vi "BM_electrochem_cell_rinse_cycle_subVI_v2.vi"(0 "Sample Volume":dbl=10.0, 1 "Pump Parameters":T1={"Speed 1"="150", "Speed 2"="250", "Speed 3"="450", "Speed 4"="250", "UW/Sample"="5", "Sparge"="2", "Std"="4", "Waste"="15", "Air"="14", "Milli-Q"="1", "H2SO4"="6", "NaOH"="3", "Catalyst"="7", "Cell (H+ side)"="8", "Cell (sample side)"="9", "NaCl"="11"}, 5 "N cell rinses":i32=3, 7 "N syringe rinses":i32=3, 9 "Extra Milli-Q (ml)":dbl=2.0, 11 "step to ml":dbl=1920.0, 12 "COM Port":refnum<visa-resource-name>="COM12", 14 "Total Vol. (mL)":dbl=12.0) -> ()   [LabVIEW 2021]
panel:
  out "Full Command":string="V450O1P38400O15D38400"
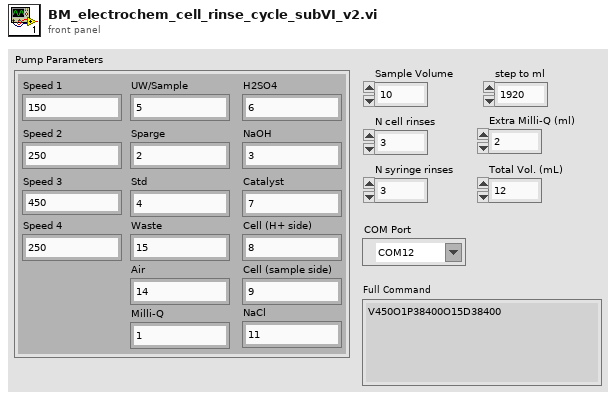
[diagram p1: front panel]
types:
  T1 = cluster{"Speed 1":string, "Speed 2":string, "Speed 3":string, "Speed 4":string, "UW/Sample":string, "Sparge":string, "Std":string, "Waste":string, "Air":string, "Milli-Q":string, "H2SO4":string, "NaOH":string, "Catalyst":string, "Cell (H+ side)":string, "Cell (sample side)":string, "NaCl":string}
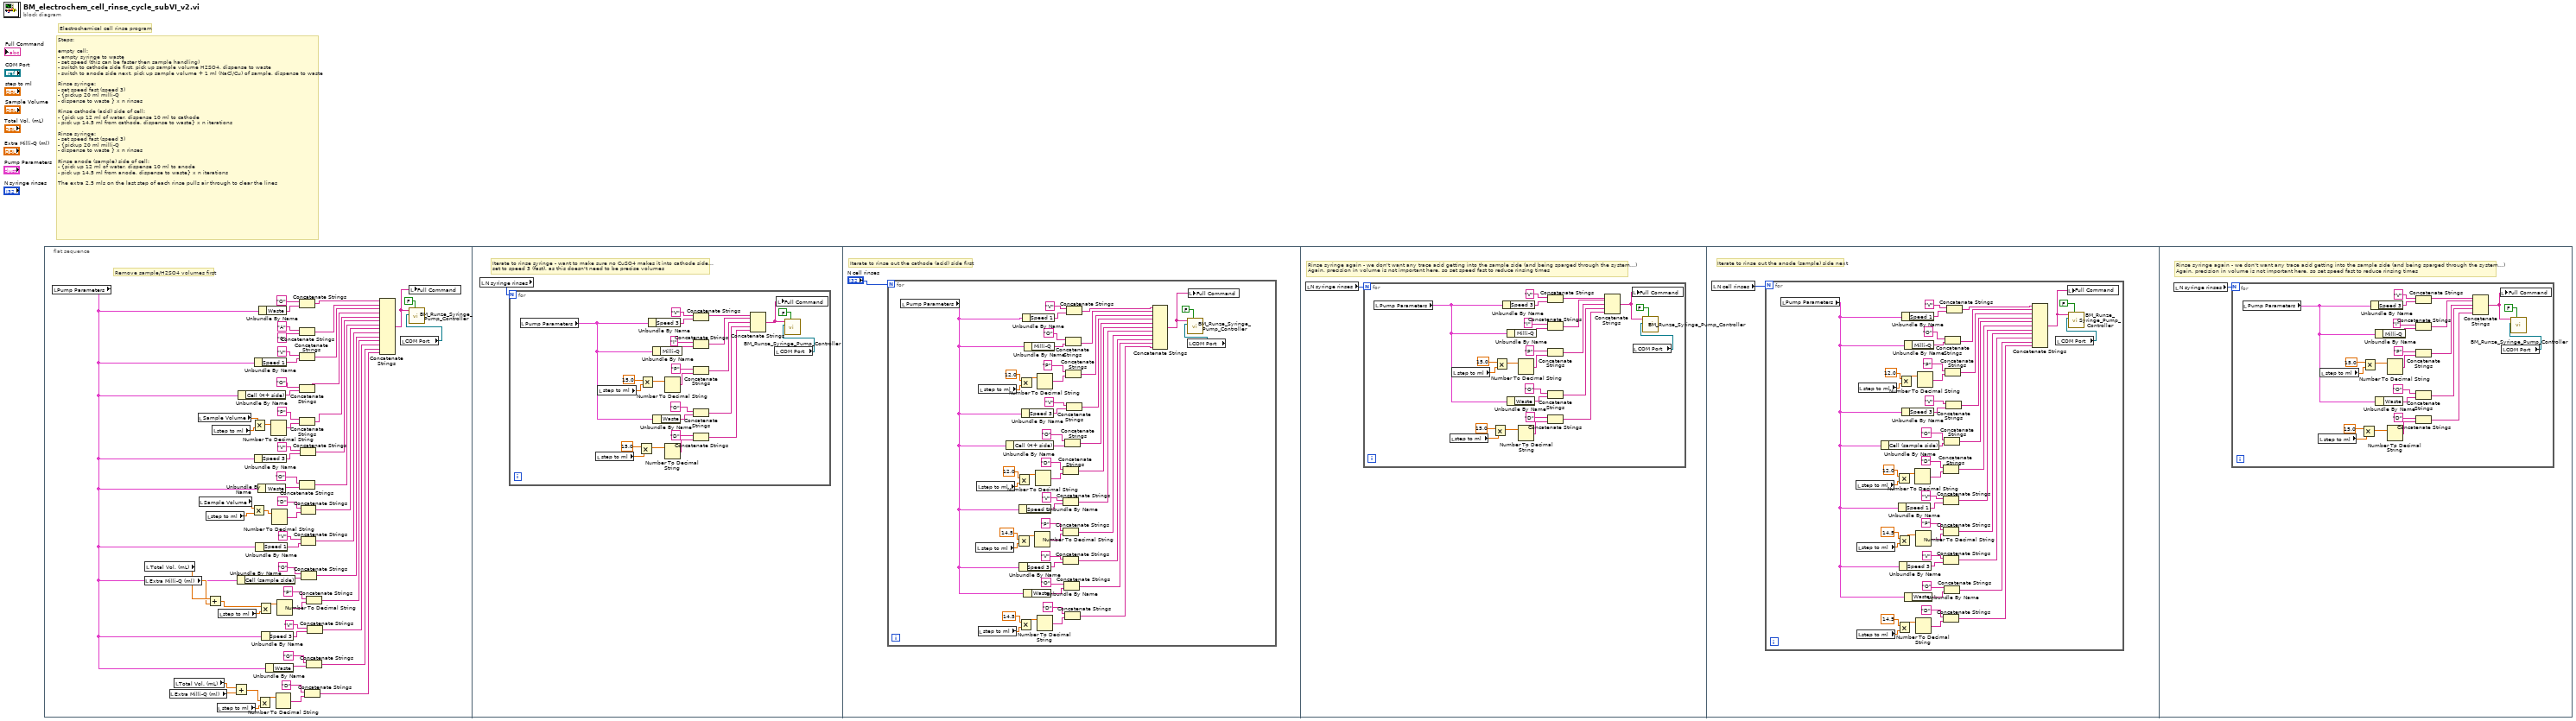
[diagram p0: block diagram]
diagram:
  # "Steps:\n\nempty cell:\n- empty syringe to waste\n- set speed (this can be faster then sample handling)\n- switch to cathode side first, pick up sample volume H2SO4, dispense to waste\n- switch to anode side next, pick up sample volume + 1 ml (NaCl/Cu) of sample, dispense to waste\n\nRinse syringe:\n- set speed fast (speed 3)\n- {pickup 20 ml milli-Q\n- dispense to waste } x n rinses\n\nRinse cathode (acid) side of cell:\n- {pick up 12 ml of water, dispense 10 ml to cathode\n- pick up 14.5 ml from cathode, dispense to waste} x n iterations\n\nRinse syringe:\n- set speed fast (speed 3)\n- {pickup 20 ml milli-Q\n- dispense to waste } x n rinses\n\nRinse anode (sample) side of cell:\n- {pick up 12 ml of water, dispense 10 ml to anode\n- pick up 14.5 ml from anode, dispense to waste} x n iterations\n\nThe extra 2.5 mls on the last step of each rinse pulls air through to clear the lines"
  # "Electrochemical cell rinse program"
  n1 = flat-sequence {
    frame #0 {
      # "Remove sample/H2SO4 volumes first"
      n2 = local read "Pump Parameters"() -> (w1:T1)
      n3 = local read "Extra Milli-Q (ml)"() -> (w30:dbl)
      n4 = local read "Total Vol. (mL)"() -> (w31:dbl)
      n5 = local read "Extra Milli-Q (ml)"() -> (w29:dbl)
      n6 = local read "Total Vol. (mL)"() -> (w19:dbl)
      n7 = local read "Sample Volume"() -> (w56:dbl)
      n8 = local read "Sample Volume"() -> (w21:dbl)
      n9 = local read "step to ml"() -> (w22:dbl)
      n10 = Add(x=w31, y=w30) -> (x+y=w27:dbl)
      n11 = local read "step to ml"() -> (w57:dbl)
      n12 = local read "step to ml"() -> (w52:dbl)
      n13 = local read "step to ml"() -> (w54:dbl)
      n14 = Add(x=w19, y=w29) -> (x+y=w18:dbl)
      n15 = Unbundle By Name(w1) -> ("Cell (sample side)"=w45:string)
      n16 = Unbundle By Name(w1) -> ("Cell (H+ side)"=w49:string)
      n17 = Multiply(x=w21, y=w22) -> (x*y=w20:dbl)
      n18 = Multiply(x=w56, y=w57) -> (x*y=w58:dbl)
      n19 = Unbundle By Name(w1) -> ("Speed 1"=w17:string)
      n20 = Unbundle By Name(w1) -> ("Speed 3"=w15:string)
      n21 = Unbundle By Name(w1) -> ("Speed 1"=w13:string)
      n22 = Multiply(x=w18, y=w52) -> (x*y=w53:dbl)
      n23 = Unbundle By Name(w1) -> ("Waste"=w25:string)
      n24 = Multiply(x=w27, y=w54) -> (x*y=w55:dbl)
      n25 = Unbundle By Name(w1) -> ("Waste"=w61:string)
      n26 = Unbundle By Name(w1) -> ("Speed 3"=w11:string)
      n27 = Unbundle By Name(w1) -> ("Waste"=w41:string)
      n28 = Number To Decimal String(number=w58) -> (decimal integer string=w47:string)  [unwired: 1 out]
      n29 = Number To Decimal String(number=w20) -> (decimal integer string=w23:string)  [unwired: 1 out]
      n30 = Number To Decimal String(number=w53) -> (decimal integer string=w39:string)  [unwired: 1 out]
      n31 = Number To Decimal String(number=w55) -> (decimal integer string=w43:string)  [unwired: 1 out]
      n32 = Concatenate Strings("O", w25) -> (w9:string)
      n33 = Concatenate Strings("O", w61) -> (w38:string)
      n34 = Concatenate Strings("A", "0") -> (w37:string)
      n35 = Concatenate Strings("V", w17) -> (w36:string)
      n36 = Concatenate Strings("O", w49) -> (w35:string)
      n37 = Concatenate Strings("P", w47) -> (w34:string)
      n38 = Concatenate Strings("V", w15) -> (w10:string)
      n39 = Concatenate Strings("D", w23) -> (w8:string)
      n40 = Concatenate Strings("V", w13) -> (w7:string)
      n41 = Concatenate Strings("O", w45) -> (w6:string)
      n42 = Concatenate Strings("D", w39) -> (w2:string)
      n43 = Concatenate Strings("P", w43) -> (w5:string)
      n44 = Concatenate Strings("O", w41) -> (w3:string)
      n45 = Concatenate Strings("V", w11) -> (w4:string)
      n46 = Concatenate Strings(w38, w37, w36, w35, w34, w10, w9, w8, w7, w6, w5, w4, w3, w2) -> (w33:string)
      n47 = local read "COM Port"() -> (w32:refnum<visa-resource-name>)
      n48 = call "BM_Runze_Syringe_Pump_Controller.vi"("Initialize Plunger?"=FALSE ("Initialize?"), "COM Port (Runze)"=w32, "Enter Command"=w33) -> ()  [unwired: 6 in, 3 out]
      n49 = local write "Full Command"(w33) -> ()
    }
    frame #1 {
      # "Iterate to rinse syringe - want to make sure no CuSO4 makes it into cathode side... \nset to speed 3 (fast), as this doesn't need to be precise volumes"
      n50 = local read "N syringe rinses"() -> (w63:i32)
      n51 = for {
        N: w63 -> [_]
        n52 = local read "Pump Parameters"() -> (w70:T1)
        n53 = local read "step to ml"() -> (w71:dbl)
        n54 = local read "step to ml"() -> (w82:dbl)
        n55 = Multiply(x=15.0, y=w71) -> (x*y=w74:dbl)
        n56 = Multiply(x=15.0, y=w82) -> (x*y=w83:dbl)
        n57 = Unbundle By Name(w70) -> ("Speed 3"=w78:string)
        n58 = Unbundle By Name(w70) -> ("Milli-Q"=w85:string)
        n59 = Unbundle By Name(w70) -> ("Waste"=w76:string)
        n60 = Number To Decimal String(number=w83) -> (decimal integer string=w80:string)  [unwired: 1 out]
        n61 = Number To Decimal String(number=w74) -> (decimal integer string=w73:string)  [unwired: 1 out]
        n62 = Concatenate Strings("V", w78) -> (w69:string)
        n63 = Concatenate Strings("I", w85) -> (w68:string)
        n64 = Concatenate Strings("P" ("string"), w80) -> (w67:string)
        n65 = Concatenate Strings("O", w76) -> (w66:string)
        n66 = Concatenate Strings("D" ("string"), w73) -> (w65:string)
        n67 = Concatenate Strings(w69, w68, w67, w66, w65) -> (w86:string)
        n68 = local read "COM Port"() -> (w87:refnum<visa-resource-name>)
        n69 = local write "Full Command"(w86) -> ()
        n70 = call "BM_Runze_Syringe_Pump_Controller.vi"("Initialize Plunger?"=FALSE ("Initialize?"), "COM Port (Runze)"=w87, "Enter Command"=w86) -> ()  [unwired: 6 in, 3 out]
      }
    }
    frame #2 {
      # "Iterate to rinse out the cathode (acid) side first"
      n71 = for {
        N: "N cell rinses" -> [_]
        n72 = local read "Pump Parameters"() -> (w93:T1)
        n73 = local read "step to ml"() -> (w130:dbl)
        n74 = local read "step to ml"() -> (w133:dbl)
        n75 = local read "step to ml"() -> (w127:dbl)
        n76 = local read "step to ml"() -> (w136:dbl)
        n77 = Unbundle By Name(w93) -> ("Cell (H+ side)"=w98:string)
        n78 = Multiply(x=14.5, y=w130) -> (x*y=w131:dbl)
        n79 = Multiply(x=12.0, y=w133) -> (x*y=w134:dbl)
        n80 = Multiply(x=14.5, y=w127) -> (x*y=w128:dbl)
        n81 = Multiply(x=12.0, y=w136) -> (x*y=w137:dbl)
        n82 = Unbundle By Name(w93) -> ("Speed 1"=w109:string)
        n83 = Unbundle By Name(w93) -> ("Speed 3"=w90:string)
        n84 = Unbundle By Name(w93) -> ("Speed 3"=w91:string)
        n85 = Unbundle By Name(w93) -> ("Speed 1"=w111:string)
        n86 = Unbundle By Name(w93) -> ("Waste"=w96:string)
        n87 = Unbundle By Name(w93) -> ("Milli-Q"=w124:string)
        n88 = Number To Decimal String(number=w131) -> (decimal integer string=w117:string)  [unwired: 1 out]
        n89 = Number To Decimal String(number=w134) -> (decimal integer string=w119:string)  [unwired: 1 out]
        n90 = Number To Decimal String(number=w128) -> (decimal integer string=w115:string)  [unwired: 1 out]
        n91 = Number To Decimal String(number=w137) -> (decimal integer string=w122:string)  [unwired: 1 out]
        n92 = Concatenate Strings("P", w117) -> (w100:string)
        n93 = Concatenate Strings("V", w90) -> (w99:string)
        n94 = Concatenate Strings("D", w119) -> (w102:string)
        n95 = Concatenate Strings("V", w109) -> (w101:string)
        n96 = Concatenate Strings("O", w96) -> (w95:string)
        n97 = Concatenate Strings("O", w98) -> (w103:string)
        n98 = Concatenate Strings("D", w115) -> (w94:string)
        n99 = Concatenate Strings("O", w124) -> (w106:string)
        n100 = Concatenate Strings("P", w122) -> (w105:string)
        n101 = Concatenate Strings("V", w91) -> (w104:string)
        n102 = Concatenate Strings("V", w111) -> (w107:string)
        n103 = Concatenate Strings(w107, w106, w105, w104, w103, w102, w101, w100, w99, w95, w94) -> (w113:string)
        n104 = local read "COM Port"() -> (w114:refnum<visa-resource-name>)
        n105 = call "BM_Runze_Syringe_Pump_Controller.vi"("Initialize Plunger?"=FALSE ("Initialize?"), "COM Port (Runze)"=w114, "Enter Command"=w113) -> ()  [unwired: 6 in, 3 out]
        n106 = local write "Full Command"(w113) -> ()
      }
    }
    frame #3 {
      # "Rinse syringe again - we don't want any trace acid getting into the sample side (and being sparged through the system...)\nAgain, precision in volume is not important here, so set speed fast to reduce rinsing times"
      n107 = local read "N syringe rinses"() -> (w139:i32)
      n108 = for {
        N: w139 -> [_]
        n109 = local read "Pump Parameters"() -> (w146:T1)
        n110 = local read "step to ml"() -> (w147:dbl)
        n111 = local read "step to ml"() -> (w158:dbl)
        n112 = Multiply(x=15.0, y=w147) -> (x*y=w150:dbl)
        n113 = Multiply(x=15.0, y=w158) -> (x*y=w159:dbl)
        n114 = Unbundle By Name(w146) -> ("Speed 3"=w154:string)
        n115 = Unbundle By Name(w146) -> ("Milli-Q"=w161:string)
        n116 = Unbundle By Name(w146) -> ("Waste"=w152:string)
        n117 = Number To Decimal String(number=w159) -> (decimal integer string=w156:string)  [unwired: 1 out]
        n118 = Number To Decimal String(number=w150) -> (decimal integer string=w149:string)  [unwired: 1 out]
        n119 = Concatenate Strings("V", w154) -> (w145:string)
        n120 = Concatenate Strings("I", w161) -> (w144:string)
        n121 = Concatenate Strings("P" ("string"), w156) -> (w143:string)
        n122 = Concatenate Strings("O", w152) -> (w142:string)
        n123 = Concatenate Strings("D" ("string"), w149) -> (w141:string)
        n124 = Concatenate Strings(w145, w144, w143, w142, w141) -> (w162:string)
        n125 = local write "Full Command"(w162) -> ()
        n126 = local read "COM Port"() -> (w163:refnum<visa-resource-name>)
        n127 = call "BM_Runze_Syringe_Pump_Controller.vi"("Initialize Plunger?"=FALSE ("Initialize?"), "COM Port (Runze)"=w163, "Enter Command"=w162) -> ()  [unwired: 6 in, 3 out]
      }
    }
    frame #4 {
      # "Iterate to rinse out the anode (sample) side next"
      n128 = local read "N cell rinses"() -> (w165:i32)
      n129 = for {
        N: w165 -> [_]
        n130 = local read "Pump Parameters"() -> (w169:T1)
        n131 = local read "step to ml"() -> (w209:dbl)
        n132 = local read "step to ml"() -> (w206:dbl)
        n133 = local read "step to ml"() -> (w203:dbl)
        n134 = local read "step to ml"() -> (w212:dbl)
        n135 = Unbundle By Name(w169) -> ("Cell (sample side)"=w196:string)
        n136 = Multiply(x=12.0, y=w209) -> (x*y=w210:dbl)
        n137 = Multiply(x=14.5, y=w206) -> (x*y=w207:dbl)
        n138 = Multiply(x=14.5, y=w203) -> (x*y=w204:dbl)
        n139 = Multiply(x=12.0, y=w212) -> (x*y=w213:dbl)
        n140 = Unbundle By Name(w169) -> ("Speed 1"=w186:string)
        n141 = Unbundle By Name(w169) -> ("Speed 3"=w166:string)
        n142 = Unbundle By Name(w169) -> ("Speed 1"=w188:string)
        n143 = Unbundle By Name(w169) -> ("Speed 3"=w167:string)
        n144 = Unbundle By Name(w169) -> ("Milli-Q"=w200:string)
        n145 = Unbundle By Name(w169) -> ("Waste"=w172:string)
        n146 = Number To Decimal String(number=w210) -> (decimal integer string=w194:string)  [unwired: 1 out]
        n147 = Number To Decimal String(number=w207) -> (decimal integer string=w192:string)  [unwired: 1 out]
        n148 = Number To Decimal String(number=w204) -> (decimal integer string=w190:string)  [unwired: 1 out]
        n149 = Number To Decimal String(number=w213) -> (decimal integer string=w198:string)  [unwired: 1 out]
        n150 = Concatenate Strings("D", w194) -> (w179:string)
        n151 = Concatenate Strings("V", w186) -> (w178:string)
        n152 = Concatenate Strings("P", w192) -> (w177:string)
        n153 = Concatenate Strings("V", w166) -> (w176:string)
        n154 = Concatenate Strings("D", w190) -> (w170:string)
        n155 = Concatenate Strings("O", w196) -> (w180:string)
        n156 = Concatenate Strings("O", w172) -> (w171:string)
        n157 = Concatenate Strings("O", w200) -> (w183:string)
        n158 = Concatenate Strings("P", w198) -> (w182:string)
        n159 = Concatenate Strings("V", w167) -> (w181:string)
        n160 = Concatenate Strings("V", w188) -> (w184:string)
        n161 = Concatenate Strings(w184, w183, w182, w181, w180, w179, w178, w177, w176, w171, w170) -> (w174:string)
        n162 = local read "COM Port"() -> (w175:refnum<visa-resource-name>)
        n163 = local write "Full Command"(w174) -> ()
        n164 = call "BM_Runze_Syringe_Pump_Controller.vi"("Initialize Plunger?"=FALSE ("Initialize?"), "COM Port (Runze)"=w175, "Enter Command"=w174) -> ()  [unwired: 6 in, 3 out]
      }
    }
    frame #5 {
      # "Rinse syringe again - we don't want any trace acid getting into the sample side (and being sparged through the system...)\nAgain, precision in volume is not important here, so set speed fast to reduce rinsing times"
      n165 = local read "N syringe rinses"() -> (w215:i32)
      n166 = for {
        N: w215 -> [_]
        n167 = local read "Pump Parameters"() -> (w222:T1)
        n168 = local read "step to ml"() -> (w223:dbl)
        n169 = local read "step to ml"() -> (w234:dbl)
        n170 = Multiply(x=15.0, y=w223) -> (x*y=w226:dbl)
        n171 = Multiply(x=15.0, y=w234) -> (x*y=w235:dbl)
        n172 = Unbundle By Name(w222) -> ("Speed 3"=w230:string)
        n173 = Unbundle By Name(w222) -> ("Milli-Q"=w237:string)
        n174 = Unbundle By Name(w222) -> ("Waste"=w228:string)
        n175 = Number To Decimal String(number=w235) -> (decimal integer string=w232:string)  [unwired: 1 out]
        n176 = Number To Decimal String(number=w226) -> (decimal integer string=w225:string)  [unwired: 1 out]
        n177 = Concatenate Strings("V", w230) -> (w221:string)
        n178 = Concatenate Strings("I", w237) -> (w220:string)
        n179 = Concatenate Strings("P" ("string"), w232) -> (w219:string)
        n180 = Concatenate Strings("O", w228) -> (w218:string)
        n181 = Concatenate Strings("D" ("string"), w225) -> (w217:string)
        n182 = Concatenate Strings(w221, w220, w219, w218, w217) -> (w238:string)
        n183 = local write "Full Command"(w238) -> ()
        n184 = local read "COM Port"() -> (w239:refnum<visa-resource-name>)
        n185 = call "BM_Runze_Syringe_Pump_Controller.vi"("Initialize Plunger?"=FALSE ("Initialize?"), "COM Port (Runze)"=w239, "Enter Command"=w238) -> ()  [unwired: 6 in, 3 out]
      }
    }
  }
